vi "myRIO_BRig_RT__Case_Exp_State_initTrial_LC_Cue1__v2.vi"(6 "input_dataTrial":u16[][](array[numeric]), 7 "input_spout":enum16{"Left", "Right"}(ring), 9 "input_dataBlock":u16[][](array[numeric]), 10 "input_dataLC":u16[](array[numeric]), 11 "input_dataCurrent":u16[](array[numeric])) -> (2 "output_LC__Cue1":bool, 3 "output_LC_led__Cue1":bool, 4 "output_dataTrial":u16[][](array[numeric]), 5 "output_dataCurrent":u16[](array[numeric]))   [LabVIEW 2014]
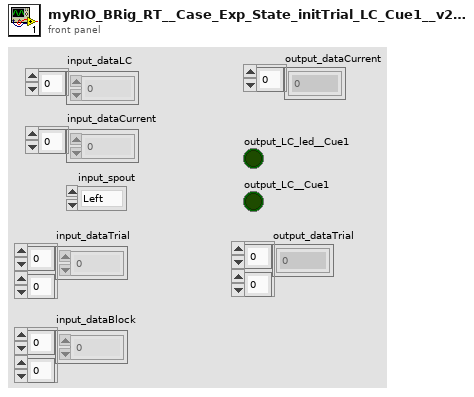
[diagram p1: front panel]
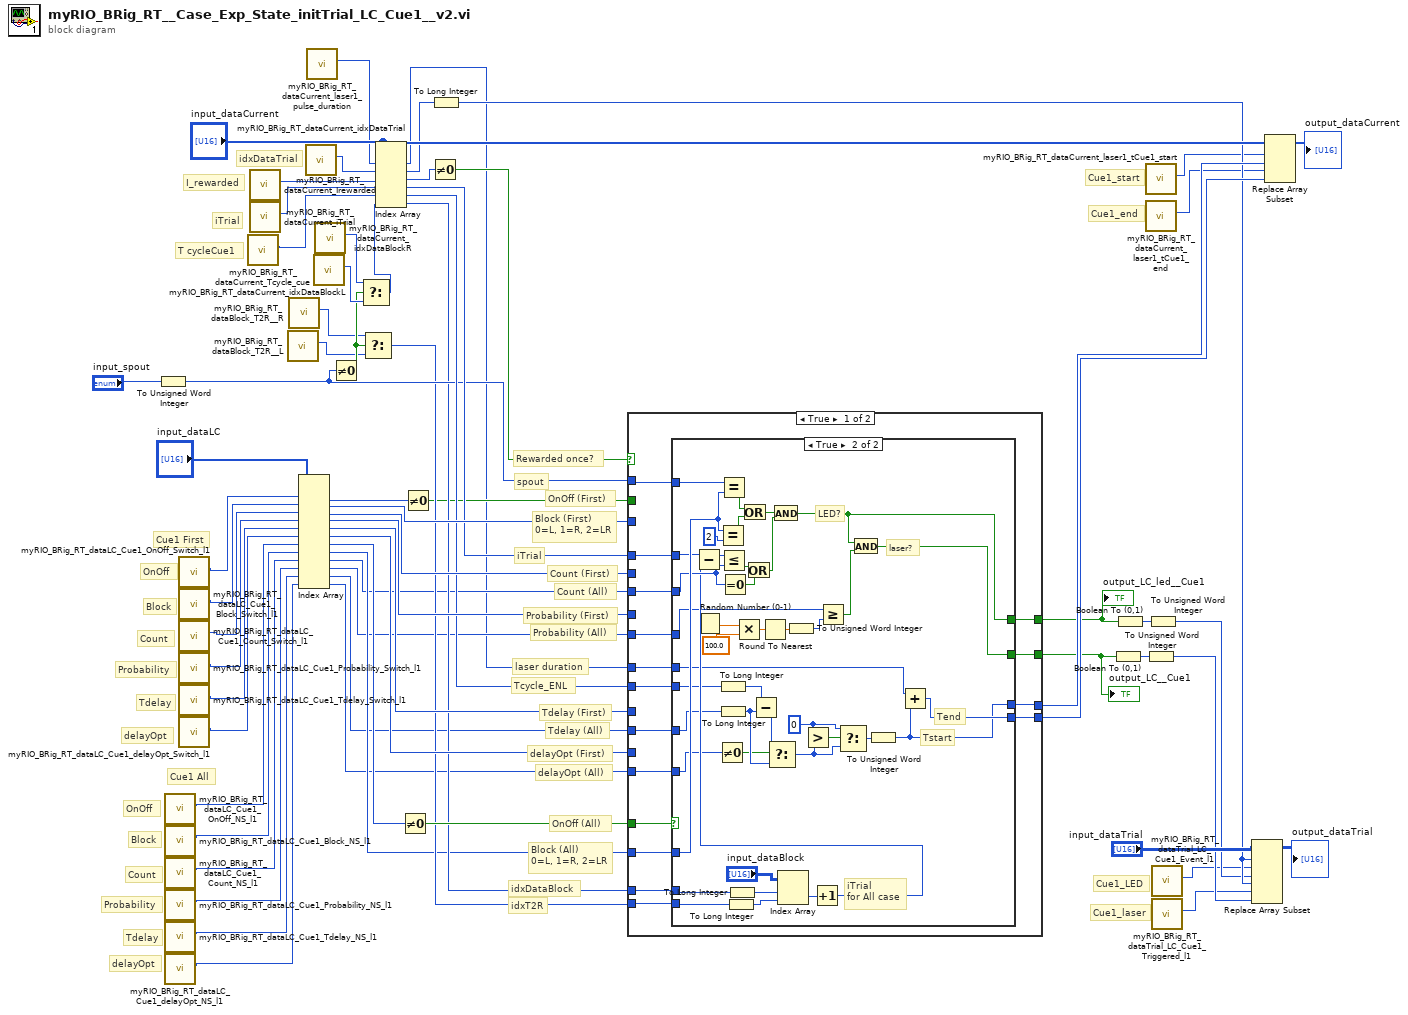
[diagram p0: block diagram]
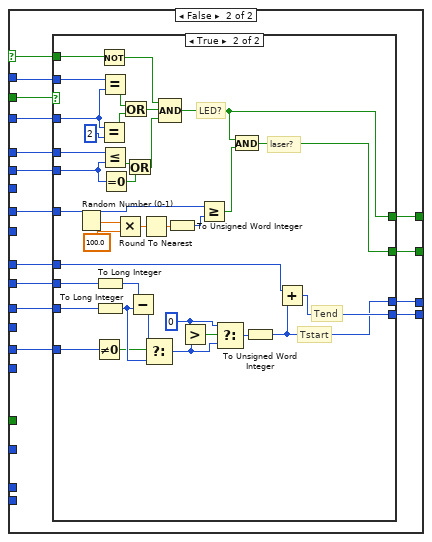
[diagram p3: hidden frame]
diagram:
  # "delayOpt (All)"
  # "Tdelay (All)"
  # "Probability (All)"
  # "Count (All)"
  # "Block (All)\n0=L, 1=R, 2=LR"
  # "idxT2R"
  # "idxDataBlock"
  # "OnOff (All)"
  # "delayOpt"
  # "Count"
  # "Tdelay"
  # "Probability"
  # "OnOff"
  # "Block"
  # "Cue1 All"
  # "Tdelay (First)"
  # "delayOpt (First)"
  # "Tcycle_ENL"
  # "laser duration"
  # "Probability (First)"
  # "Count (First)"
  # "iTrial"
  # "Block (First)\n0=L, 1=R, 2=LR"
  # "spout"
  # "Rewarded once?"
  # "OnOff (First)"
  # "iTrial"
  # "Cue1_LED"
  # "Cue1_laser"
  # "idxDataTrial"
  # "Cue1_end"
  # "Cue1_start"
  # "delayOpt"
  # "T cycleCue1"
  # "Tdelay"
  # "I_rewarded"
  # "Cue1 First"
  # "Probability"
  # "Count"
  # "Block"
  # "OnOff"
  n1 = To Unsigned Word Integer(number="input_spout") -> (unsigned 16bit integer=w35:u16)
  n2 = call "myRIO_BRig_RT_dataLC_Cue1_OnOff_NS_l1.vi"() -> ("output_Cue1_OnOff_NS_l1"=w8:i32)  [unwired: 11 in]
  n3 = call "myRIO_BRig_RT_dataLC_Cue1_Block_NS_l1.vi"() -> ("output_Cue1_Block_NS_l1"=w9:i32)  [unwired: 11 in]
  n4 = call "myRIO_BRig_RT_dataLC_Cue1_Count_NS_l1.vi"() -> ("output_Cue1_Count_NS_l1"=w10:i32)  [unwired: 11 in]
  n5 = call "myRIO_BRig_RT_dataLC_Cue1_Probability_NS_l1.vi"() -> ("output_Cue1_l1_All_Probability"=w11:i32)  [unwired: 11 in]
  n6 = call "myRIO_BRig_RT_dataLC_Cue1_Tdelay_NS_l1.vi"() -> ("output_Cue1_Tdelay_NS_l1"=w12:i32)  [unwired: 11 in]
  n7 = call "myRIO_BRig_RT_dataLC_Cue1_delayOpt_NS_l1.vi"() -> ("output_Cue1_delayOpt_NS_l1"=w13:i32)  [unwired: 11 in]
  n8 = call "myRIO_BRig_RT_dataLC_Cue1_OnOff_Switch_l1.vi"() -> ("output_Cue1_OnOff_Switch_l1"=w14:i32)  [unwired: 11 in]
  n9 = call "myRIO_BRig_RT_dataLC_Cue1_Block_Switch_l1.vi"() -> ("output_Cue1_Block_Switch_l1"=w15:i32)  [unwired: 11 in]
  n10 = call "myRIO_BRig_RT_dataLC_Cue1_Count_Switch_l1.vi"() -> ("output_Cue1_Count_Switch_l1"=w16:i32)  [unwired: 11 in]
  n11 = call "myRIO_BRig_RT_dataLC_Cue1_Probability_Switch_l1.vi"() -> ("output_Cue1_Probability_Switch_l1"=w17:i32)  [unwired: 11 in]
  n12 = call "myRIO_BRig_RT_dataLC_Cue1_Tdelay_Switch_l1.vi"() -> ("output_Cue1_Tdelay_Switch_l1"=w18:i32)  [unwired: 11 in]
  n13 = call "myRIO_BRig_RT_dataLC_Cue1_delayOpt_Switch_l1.vi"() -> ("output_Cue1_delayOpt_Switch_l1"=w19:i32)  [unwired: 11 in]
  n14 = call "myRIO_BRig_RT_dataCurrent_Tcycle_cue.vi"() -> ("output_Tcycle_cue"=w7:i32)  [unwired: 11 in]
  n15 = call "myRIO_BRig_RT_dataCurrent_Irewarded.vi"() -> ("output_I_rewarded"=w58:i32)  [unwired: 11 in]
  n16 = call "myRIO_BRig_RT_dataCurrent_iTrial.vi"() -> ("output_iTrial"=w39:i32)  [unwired: 11 in]
  n17 = call "myRIO_BRig_RT_dataBlock_T2R__L.vi"() -> ("output_T2R__L"=w29:i32)  [unwired: 11 in]
  n18 = call "myRIO_BRig_RT_dataBlock_T2R__R.vi"() -> ("output_T2R__R"=w30:i32)  [unwired: 11 in]
  n19 = Index Array(array="input_dataLC", index #1=w14, index #2=w15, index #3=w16, index #4=w17, index #5=w18, index #6=w19, index #7=w8, index #8=w9, index #9=w10, index #10=w11, index #11=w12, index #12=w13) -> (element #1=w64:u16, element #2=w61:u16, element #3=w62:u16, element #4=w63:u16, element #5=w57:u16, element #6=w56:u16, element #7=w37:u16, element #8=w26:u16, element #9=w25:u16, element #10=w24:u16, element #11=w23:u16, element #12=w22:u16)
  n20 = call "myRIO_BRig_RT_dataCurrent_idxDataTrial.vi"() -> ("output_idxDataTrial"=w45:i32)  [unwired: 11 in]
  n21 = call "myRIO_BRig_RT_dataCurrent_laser1_pulse_duration.vi"() -> ("output_laser1_pulse_duration"=w2:i32)  [unwired: 11 in]
  n22 = call "myRIO_BRig_RT_dataCurrent_idxDataBlockL.vi"() -> ("output_idxDataBlock__L"=w34:i32)  [unwired: 11 in]
  n23 = call "myRIO_BRig_RT_dataCurrent_idxDataBlockR.vi"() -> ("output_idxDataBlock__R"=w33:i32)  [unwired: 11 in]
  n24 = Not Equal To 0?(x=w35) -> (x != 0?=w31:bool)
  n25 = Select(t=w33, s=w31, f=w34) -> (s? t:f=w32:i32)
  n26 = Select(t=w30, s=w31, f=w29) -> (s? t:f=w27:i32)
  n27 = Index Array(array="input_dataCurrent", index #1=w2, index #2=w45, index #3=w58, index #4=w39, index #5=w7, index #6=w32) -> (element #1=w1:u16, element #2=w44:u16, element #3=w59:u16, element #4=w38:u16, element #5=w40:u16, element #6=w28:u16)
  n28 = Not Equal To 0?(x=w37) -> (x != 0?=w36:bool)
  n29 = Not Equal To 0?(x=w64) -> (x != 0?=w20:bool)
  n30 = Not Equal To 0?(x=w59) -> (x != 0?=w21:bool)
  n31 = To Long Integer(number=w44) -> (32bit integer=w43:i32)
  n32 = case shown="True" w21 {
    selector: w21 -> [_ w125]
    tunnel: w61 -> [_ w137]
    tunnel: w62 -> [_ w128]
    tunnel: w63 -> [_ w135]
    tunnel: [w78 w133] -> w48
    tunnel: [w79 w134] -> w50
    tunnel: w35 -> [w81 w138]
    tunnel: w57 -> [_ w130]
    tunnel: w56 -> [_ w131]
    tunnel: w40 -> [w74 w127]
    tunnel: w1 -> [w75 w126]
    tunnel: [w76 w129] -> w53
    tunnel: [w77 w132] -> w52
    tunnel: w38 -> [w80 w136]
    tunnel: w36 -> [w66 _]
    tunnel: w27 -> [w73 _]
    tunnel: w28 -> [w72 _]
    tunnel: w26 -> [w71 _]
    tunnel: w25 -> [w70 _]
    tunnel: w24 -> [w69 _]
    tunnel: w23 -> [w68 _]
    tunnel: w22 -> [w67 _]
    tunnel: w20 -> [_ w124]
    frame True {
      n33 = case shown="True" w66 {
        tunnel: w81 -> [_ w122]
        tunnel: w80 -> [_ w101]
        tunnel: [_ w96] -> w79
        tunnel: [_ w113] -> w78
        tunnel: [_ w87] -> w77
        tunnel: [_ w86] -> w76
        tunnel: w75 -> [_ w85]
        tunnel: w74 -> [_ w84]
        tunnel: w73 -> [_ w107]
        tunnel: w72 -> [_ w109]
        tunnel: w71 -> [_ w104]
        tunnel: w70 -> [_ w103]
        tunnel: w69 -> [_ w99]
        tunnel: w68 -> [_ w83]
        tunnel: w67 -> [_ w82]
        frame False {
        }
        frame True {
          w93 = 0 ("x")
          # "Tstart"
          # "Tend"
          # "iTrial\nfor All case"
          # "laser?"
          # "LED?"
          n34 = Random Number (0-1)() -> (number: 0 to 1=w119:dbl)
          n35 = Not Equal To 0?(x=w82) -> (x != 0?=w90:bool)
          n36 = Equal?(x=w104, y=u16 2) -> (x = y?=w120:bool)
          n37 = To Long Integer(number=w84) -> (32bit integer=w88:i32)
          n38 = To Long Integer(number=w83) -> (32bit integer=w91:i32)
          n39 = Equal?(x=w122, y=w104) -> (x = y?=w121:bool)
          n40 = Equal To 0?(x=w103) -> (x = 0?=w111:bool)
          n41 = To Long Integer(number=w107) -> (32bit integer=w106:i32)
          n42 = To Long Integer(number=w109) -> (32bit integer=w108:i32)
          n43 = Multiply(x=w119, y=100.0) -> (x*y=w118:dbl)
          n44 = Or(x=w121, y=w120) -> (x .or. y?=w98:bool)
          n45 = Subtract(x=w88, y=w91) -> (x-y=w89:i32)
          n46 = Round To Nearest(number=w118) -> (nearest integer value=w117:dbl)
          n47 = Select(t=w89, s=w90, f=w91) -> (s? t:f=w94:i32)
          n48 = Index Array(array="input_dataBlock", index (row)=w108, index (col)=w106) -> (element=w105:u16)
          n49 = To Unsigned Word Integer(number=w117) -> (unsigned 16bit integer=w115:u16)
          n50 = Greater?(x=w93, y=w94) -> (0:w92:bool)
          n51 = Increment(x=w105) -> (x+1=w102:u16)
          n52 = Subtract(x=w101, y=w102) -> (x-y=w100:u16)
          n53 = Less Or Equal?(x=w100, y=w103) -> (x <= y?=w112:bool)
          n54 = Or(x=w112, y=w111) -> (x .or. y?=w97:bool)
          n55 = And(x=w98, y=w97) -> (x .and. y?=w96:bool)
          n56 = Greater Or Equal?(x=w99, y=w115) -> (x >= y?=w114:bool)
          n57 = Select(t=w93, s=w92, f=w94) -> (s? t:f=w95:i32)
          n58 = And(x=w96, y=w114) -> (x .and. y?=w113:bool)
          n59 = To Unsigned Word Integer(number=w95) -> (unsigned 16bit integer=w86:u16)
          n60 = Add(x=w85, y=w86) -> (x+y=w87:u16)
        }
      }
    }
    frame False {
      n61 = case shown="True" w124 {
        tunnel: w138 -> [_ w173]
        tunnel: w137 -> [_ w172]
        tunnel: w136 -> [_ w171]
        tunnel: w135 -> [_ w164]
        tunnel: [_ w159] -> w134
        tunnel: [_ w158] -> w133
        tunnel: [_ w140] -> w132
        tunnel: w131 -> [_ w144]
        tunnel: w130 -> [_ w143]
        tunnel: [_ w139] -> w129
        tunnel: w128 -> [_ w157]
        tunnel: w127 -> [_ w142]
        tunnel: w126 -> [_ w141]
        tunnel: w125 -> [_ w153]
        frame False {
        }
        frame True {
          w150 = 0 ("x")
          # "Tstart"
          # "Tend"
          # "laser?"
          # "LED?"
          n62 = Random Number (0-1)() -> (number: 0 to 1=w168:dbl)
          n63 = Not Equal To 0?(x=w144) -> (x != 0?=w147:bool)
          n64 = To Long Integer(number=w142) -> (32bit integer=w145:i32)
          n65 = To Long Integer(number=w143) -> (32bit integer=w148:i32)
          n66 = Not(x=w153) -> (.not. x?=w162:bool)
          n67 = Equal?(x=w172, y=u16 2) -> (x = y?=w169:bool)
          n68 = Equal?(x=w173, y=w172) -> (x = y?=w170:bool)
          n69 = Less Or Equal?(x=w171, y=w157) -> (x <= y?=w156:bool)
          n70 = Equal To 0?(x=w157) -> (x = 0?=w155:bool)
          n71 = Multiply(x=w168, y=100.0) -> (x*y=w167:dbl)
          n72 = Or(x=w170, y=w169) -> (x .or. y?=w161:bool)
          n73 = Or(x=w156, y=w155) -> (x .or. y?=w154:bool)
          n74 = Subtract(x=w145, y=w148) -> (x-y=w146:i32)
          n75 = Round To Nearest(number=w167) -> (nearest integer value=w166:dbl)
          n76 = Select(t=w146, s=w147, f=w148) -> (s? t:f=w151:i32)
          n77 = Compound Arithmetic op=AND(w162, w161, w154) -> (w159:bool)
          n78 = To Unsigned Word Integer(number=w166) -> (unsigned 16bit integer=w163:u16)
          n79 = Greater?(x=w150, y=w151) -> (0:w149:bool)
          n80 = Greater Or Equal?(x=w164, y=w163) -> (x >= y?=w160:bool)
          n81 = Select(t=w150, s=w149, f=w151) -> (s? t:f=w152:i32)
          n82 = And(x=w159, y=w160) -> (x .and. y?=w158:bool)
          n83 = To Unsigned Word Integer(number=w152) -> (unsigned 16bit integer=w139:u16)
          n84 = Add(x=w141, y=w139) -> (x+y=w140:u16)
        }
      }
    }
  }
  "output_LC__Cue1" <- w48
  "output_LC_led__Cue1" <- w50
  n85 = Boolean To (0,1)(Boolean=w48) -> (0, 1=w49:i16)
  n86 = Boolean To (0,1)(Boolean=w50) -> (0, 1=w51:i16)
  n87 = call "myRIO_BRig_RT_dataCurrent_laser1_tCue1_start.vi"() -> ("output_laser1_tCue1_start"=w5:i32)  [unwired: 11 in]
  n88 = call "myRIO_BRig_RT_dataCurrent_laser1_tCue1_end.vi"() -> ("output_laser1_tCue1_end"=w6:i32)  [unwired: 11 in]
  n89 = To Unsigned Word Integer(number=w49) -> (unsigned 16bit integer=w41:u16)
  n90 = To Unsigned Word Integer(number=w51) -> (unsigned 16bit integer=w42:u16)
  n91 = call "myRIO_BRig_RT_dataTrial_LC_Cue1_Event_l1.vi"() -> ("output_LC_Cue1_Event_l1"=w4:i32)  [unwired: 11 in]
  n92 = call "myRIO_BRig_RT_dataTrial_LC_Cue1_Triggered_l1.vi"() -> ("output_LC_Cue1_Triggered_l1"=w3:i32)  [unwired: 11 in]
  n93 = Replace Array Subset(array="input_dataTrial", new element #1=w42, index (row) #1=w43, index (col) #1=w4, new element #2=w41, index (row) #2=w43, index (col) #2=w3) -> (→"output_dataTrial":u16[][])
  n94 = Replace Array Subset(array="input_dataCurrent", new element #1=w53, index #1=w5, new element #2=w52, index #2=w6) -> (→"output_dataCurrent":u16[])
